vi "Manual Mode - Set Configurations.vi"   [LabVIEW 2014, in "Associated Power Technologies 8500 Series.lvlib"]
uses:
  <instrlib>/Associated Power Technologies 8500 Series/Associated Power Technologies 8500 Series.lvlib
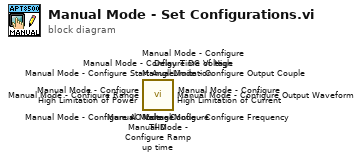
[diagram p0: block diagram]
diagram:
  n1 = call <instrlib>:"Manual Mode - Configure THD.vi"() -> ()  [unwired: 10 in, 2 out]
  n2 = call <instrlib>:"Manual Mode - Configure Delay Time of High Limitation.vi"() -> ()  [unwired: 10 in, 2 out]
  n3 = call <instrlib>:"Manual Mode - Configure High Limitation of Power.vi"() -> ()  [unwired: 10 in, 2 out]
  n4 = call <instrlib>:"Manual Mode - Configure High Limitation of Current.vi"() -> ()  [unwired: 10 in, 2 out]
  n5 = call <instrlib>:"Manual Mode - Configure Start Angle.vi"() -> ()  [unwired: 10 in, 2 out]
  n6 = call <instrlib>:"Manual Mode - Configure Ramp up time.vi"() -> ()  [unwired: 10 in, 2 out]
  n7 = call <instrlib>:"Manual Mode - Configure Frequency.vi"() -> ()  [unwired: 10 in, 2 out]
  n8 = call <instrlib>:"Manual Mode - Configure DC Voltage.vi"() -> ()  [unwired: 10 in, 2 out]
  n9 = call <instrlib>:"Manual Mode - Configure AC Voltage.vi"() -> ()  [unwired: 10 in, 2 out]
  n10 = call <instrlib>:"Manual Mode - Configure Range.vi"() -> ()  [unwired: 10 in, 2 out]
  n11 = call <instrlib>:"Manual Mode - Configure Output Waveform.vi"() -> ()  [unwired: 10 in, 2 out]
  n12 = call <instrlib>:"Manual Mode - Configure Output Couple.vi"() -> ()  [unwired: 10 in, 2 out]
